vi "dg535 error handler.vi"(2 "error in":errorcluster, 3 "check bit #":dbl min=0.0 max=6.0, 4 "command string":string, 5 "GPIB address":string="15") -> (0 "error out":errorcluster, 1 "error found":bool)   [LabVIEW 2011]
doc: "This support subVI queries the instrument's error status bits which reports an execution error .\n ERROR FOUND is set to TRUE when an out of range parameter or a delay linkage error causes an execution error . \n This subVI is used in the function subVIs after setting some or all of the instrument's functions .\n The status of ERROR FOUND is then used in the function subVIs to report an error for the parameter that caused it ."
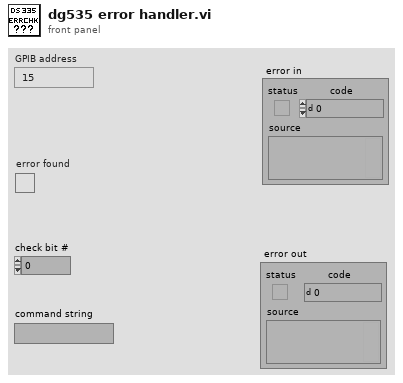
[diagram p1: front panel]
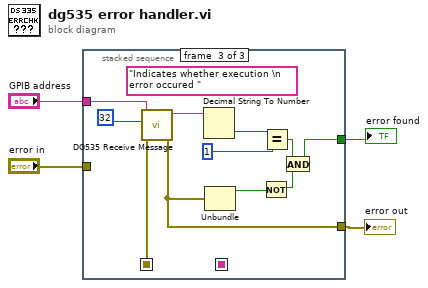
[diagram p0: block diagram]
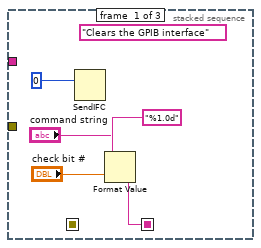
[diagram p2: hidden frame]
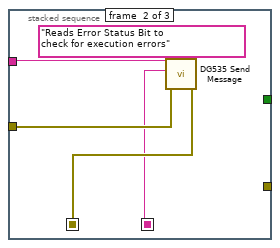
[diagram p3: hidden frame]
diagram:
  n1 = stacked-sequence {
    seq-local: [_ w12 _] -> [_ _ w24]
    seq-local: [w7 _ _] -> [_ w10 _]
    tunnel: "GPIB address" -> [_ w13 w23]
    tunnel: "error in" -> [_ w11 _]
    tunnel: [_ _ w14] -> w2
    tunnel: [_ _ w15] -> w1
    frame #0 {
      (unwired) "Clears the GPIB interface"
      n2 = SendIFC(3:0) -> ()  [unwired: 1 in, 2 out]
      n3 = Format Value(string ("")="command string", format string="%1.0d", value (0)="check bit #") -> (output string=w7:string)
    }
    frame #1 {
      (unwired) "Reads Error Status Bit to                                                    check for execution errors"
      n4 = call "DG535 Send Message.vi"("address string"=w13, "write buffer"=w10, "error in"=w11) -> ("error out"=w12:errorcluster)  [unwired: 4 in, 2 out]
    }
    frame #2 {
      (unwired) "Indicates whether execution \n          error occured "
      n5 = call "DG535 Receive Message.vi"("address string"=w23, "byte count"=32, "error in"=w24) -> ("read buffer"=w21:string, "error out"=w14:errorcluster)  [unwired: 4 in, 1 out]
      n6 = Decimal String To Number(string=w21) -> (number=w20:i32)  [unwired: 2 in, 1 out]
      n7 = Unbundle(w14) -> ("status"=w18:bool)  [unwired: 2 out]
      n8 = Not(x=w18) -> (.not. x?=w17:bool)
      n9 = Equal?(x=w20, y=1) -> (x = y?=w16:bool)
      n10 = And(x=w16, y=w17) -> (x .and. y?=w15:bool)
    }
  }
  "error out" <- w2
  "error found" <- w1
